vi "ANAL_ProtoGraph.vi"(10 "Main Data Array In":T2 {"Run Data Cluster"."Temperature B" scale=0.0..100.0; "Run Data Cluster"."Temperature A" scale=0.0..100.0}) -> (0 "Temp Graph":cluster{"Temperature A":dbl, "Numeric":i32}[](array[cluster]), 1 "Time Graph":T1(array[cluster]), 2 "Main Data Array Out":T2 {"Run Data Cluster"."Temperature B" scale=0.0..100.0; "Run Data Cluster"."Temperature A" scale=0.0..100.0}, 4 "Bin Graph":cluster{"Bin Value":i32, "Numeric":i32}[](array[cluster]))   [LabVIEW 2021]
uses:
  ANAL_Data.ctl
  XML_Cluster.ctl
  DAT_Cluster.ctl
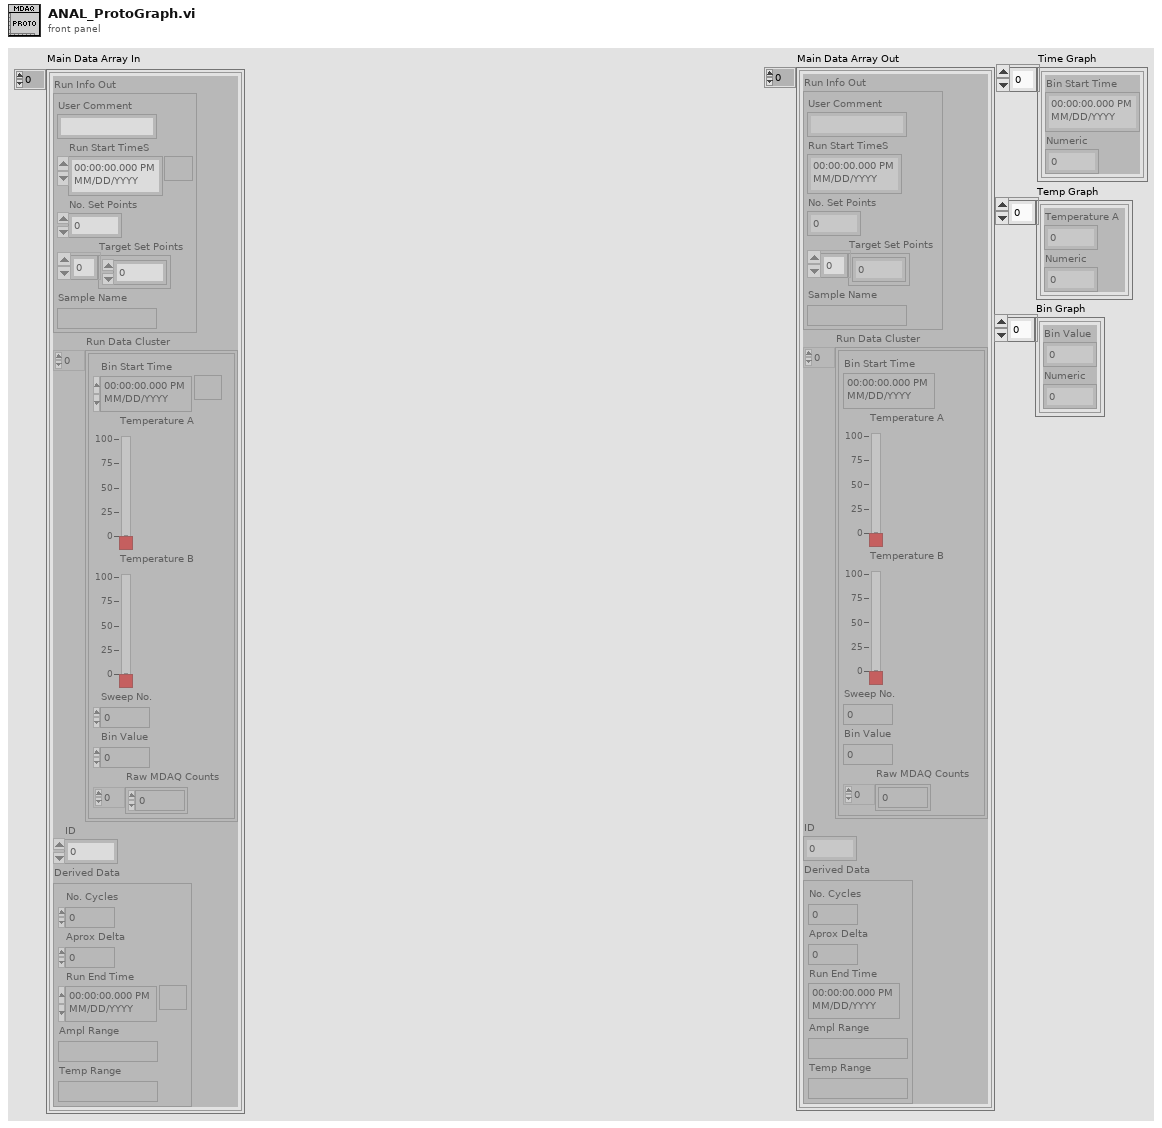
[diagram p1: front panel]
types:
  T1 = cluster{"Bin Start Time":timestamp, "Numeric":i32}[]
  T2 = typedef "ANAL_Data.ctl" = cluster{"Run Info Out":T3, "Run Data Cluster":T4, "ID":u32, "Derived Data":cluster{"No. Cycles":u32, "Aprox Delta":dbl, "Run End Time":timestamp, "Ampl Range":string, "Temp Range":string}}[]
  T3 = typedef "XML_Cluster.ctl" = cluster{"User Comment":string, "Run Start TimeS":timestamp, "No. Set Points":u32, "Target Set Points":i32[], "Sample Name":string}
  T4 = typedef "DAT_Cluster.ctl" = cluster{"Bin Start Time":timestamp, "Temperature A":dbl, "Temperature B":dbl, "Sweep No.":i32, "Bin Value":i32, "Raw MDAQ Counts":i32[]}[]
  T5 = cluster{"Run Info Out":T3, "Run Data Cluster":T4, "ID":u32, "Derived Data":cluster{"No. Cycles":u32, "Aprox Delta":dbl, "Run End Time":timestamp, "Ampl Range":string, "Temp Range":string}}
  T6 = cluster{"Bin Start Time":timestamp, "Numeric":i32}
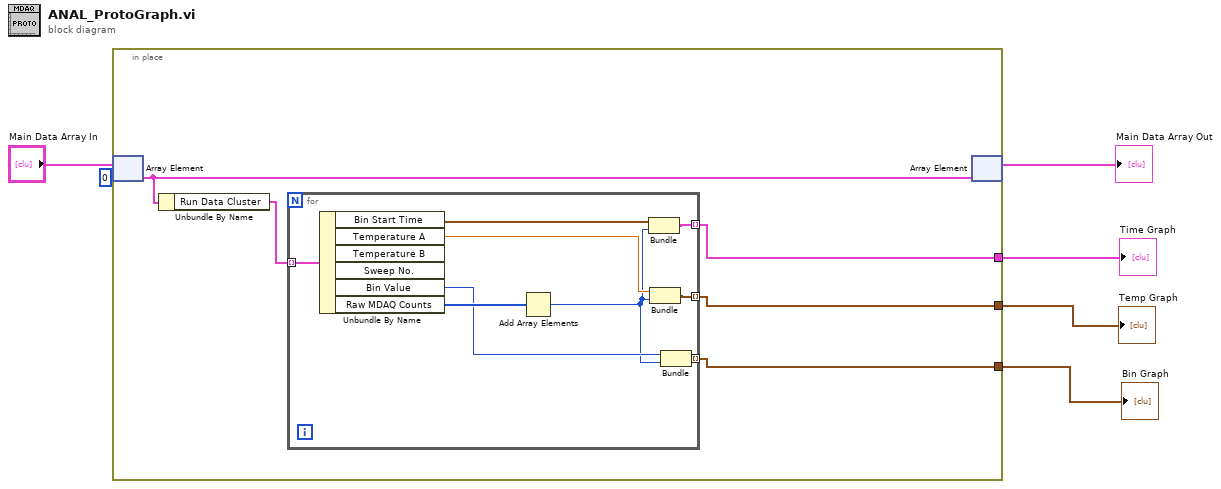
[diagram p0: block diagram]
diagram:
  n1 = in-place {
    in-place-border: [w9] -> w3
    in-place-border: [w8] -> w2
    in-place-border: [w7] -> w1
    n2 = in-place-array #1("Main Data Array In", 0) -> (w11:T5)
    n3 = Unbundle By Name(w11) -> ("Run Data Cluster"=w10:T4)
    n4 = for {
      tunnel: w10 -> [w20] mode=indexing
      tunnel: [w17] -> w9 mode=indexing
      tunnel: [w15] -> w8 mode=indexing
      tunnel: [w12] -> w7 mode=indexing
      n5 = Unbundle By Name(w20) -> ("Bin Start Time"=w19:timestamp, "Temperature A"=w16:dbl, "Bin Value"=w14:i32, "Raw MDAQ Counts"=w18:i32[])  [unwired: 2 out]
      n6 = Add Array Elements(numeric array=w18) -> (sum=w13:i32)
      n7 = Bundle("Bin Start Time"=w19, "Numeric"=w13) -> (w17:T6)  [unwired: 1 in]
      n8 = Bundle("Temperature A"=w16, "Numeric"=w13) -> (w15:cluster{"Temperature A":dbl, "Numeric":i32})  [unwired: 1 in]
      n9 = Bundle("Bin Value"=w14, "Numeric"=w13) -> (w12:cluster{"Bin Value":i32, "Numeric":i32})  [unwired: 1 in]
    }
    n10 = in-place-array #1(w11) -> (→"Main Data Array Out":T2)  [unwired: 1 out]
  }
  "Time Graph" <- w3
  "Temp Graph" <- w2
  "Bin Graph" <- w1
